vi "RT Communication Handler.vi"(8 "error in (no error)":errorcluster) -> (0 "error out":errorcluster)   [LabVIEW 2021]
uses:
  Controls/Communication Message Names.ctl
  Real-Time/Controls/Data FGV Action.ctl
  Controls/Scope & FGen Parameters.ctl
  Program Files (x86)/National Instruments/LabVIEW 2021/ProjectTemplates/Source/myRIO/Oscilloscope/myRIO v1.1/Real-Time/Controls/Wave Parameters.ctl
  Program Files (x86)/National Instruments/LabVIEW 2021/ProjectTemplates/Source/myRIO/Oscilloscope/myRIO v1.1/Real-Time/Controls/Waveform Enum.ctl
  Program Files (x86)/National Instruments/LabVIEW 2021/ProjectTemplates/Source/myRIO/Oscilloscope/myRIO v1.1/Real-Time/Controls/Channel Selector.ctl
  Controls/Time Selector.ctl
  Controls/Time Knob.ctl
  <vilib>/NI/STM/TCP/Write Meta Data (TCP Ref).vi
  <vilib>/NI/STM/TCP/Get Connection Reference (TCP).vi
  <vilib>/NI/STM/TCP/Write Meta Data (TCP Clst).vi
  <vilib>/NI/STM/TCP/Read Message (TCP).vi
  Real-Time/Controls/Global Stop.vi
  <vilib>/NI/STM/TCP/Write Message (TCP).vi
  <vilib>/NI/STM/NI STM.lvlib
panel:
  in  "Messages":T1=enum."New Settings"
  out "stop":bool
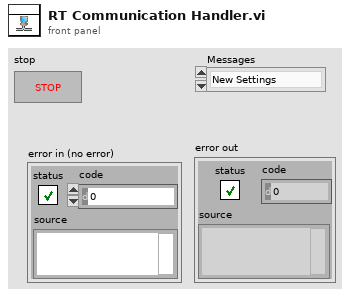
[diagram p1: front panel]
types:
  T1 = typedef "Communication Message Names.ctl" = enum16{"Status Check", "New Settings", "Measurements", "Acquire", "Params", "Initialize", "Stop"}
  T2 = typedef "Data FGV Action.ctl" = enum16{"Initialize", "Set Scope Data", "Read Scope Data", "Set FGen", "Read FGen", "Set Params"}
  T3 = typedef "Scope & FGen Parameters.ctl" = cluster{"Acquire?":bool, "Wave Parameters":T4, "Time":T7}
  T4 = typedef "Wave Parameters.ctl" = cluster{"Frequency (Hz)":dbl, "Phase offset (deg)":dbl, "Vpeak (V)":dbl, "Offset (V)":dbl, "Waveform":T5, "Channel":T6}
  T5 = typedef "Waveform Enum.ctl" = enum16{"Sine", "Square"}
  T6 = typedef "Channel Selector.ctl" = enum16{"CH0", "CH1"}
  T7 = typedef "Time Selector.ctl" = cluster{"Time/Div":T8}
  T8 = typedef "Time Knob.ctl" = dbl
  T9 = typedef "NI STM.lvlib/TCP Connection Info.ctl" = cluster{"connection ID":refnum<k5>, "meta data":T10[]}
  T10 = typedef "NI STM.lvlib/MetaDataElement.ctl" = string
  T11 = typedef "Scope Data.ctl" = cluster{"AI0":dbl[], "AI1":dbl[]}
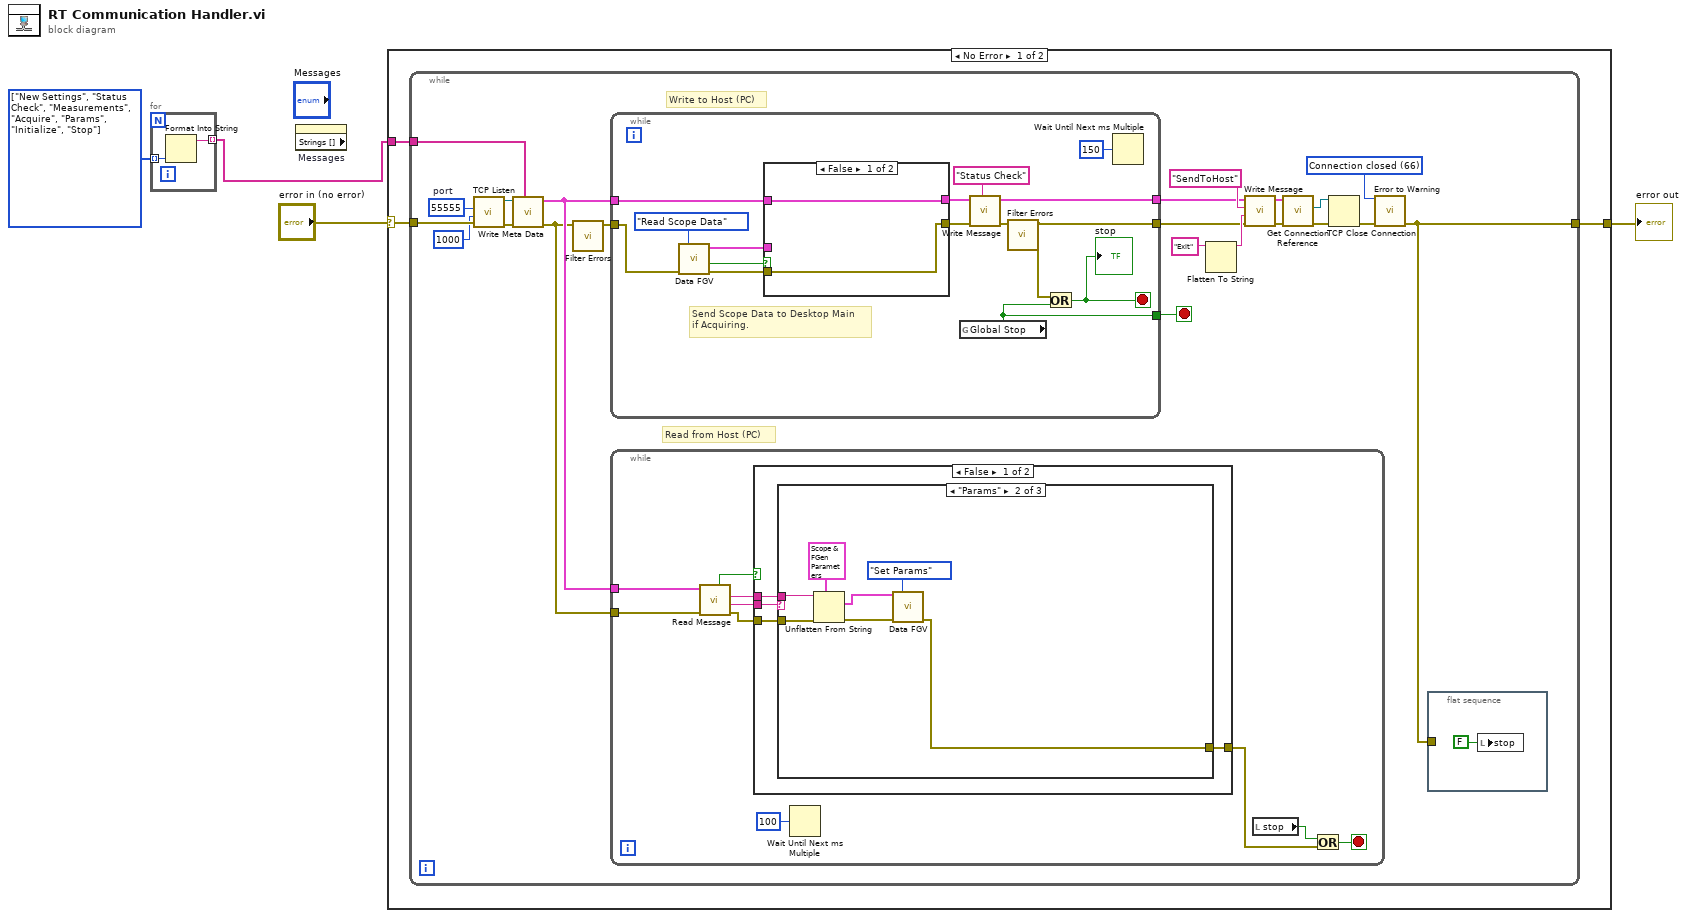
[diagram p0: block diagram]
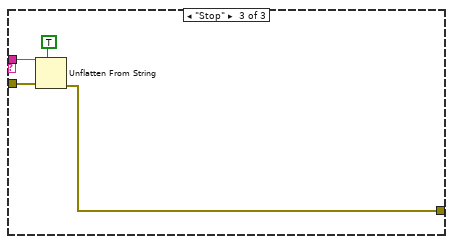
[diagram p3: hidden frame]
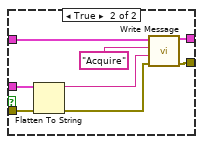
[diagram p5: hidden frame]
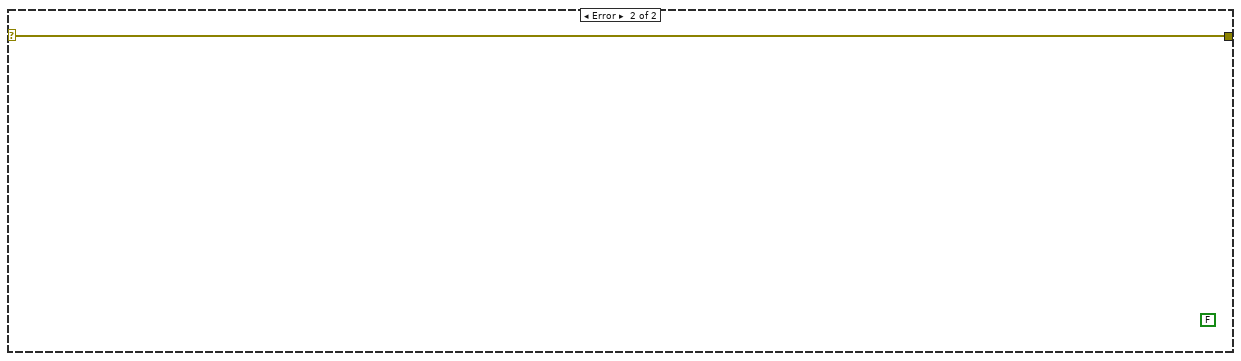
[diagram p6: hidden frame]
diagram:
  w2 = T1[] [enum."New Settings", enum."Status Check", enum."Measurements", enum."Acquire", enum."Params", enum."Initialize", enum."Stop"] items=["Status Check", "New Settings", "Measurements", "Acquire", "Params", "Initialize", "Stop"]
  n1 = for {
    tunnel: w2 -> [w6] mode=indexing
    tunnel: [w5] -> w1 mode=indexing
    n2 = Format Into String(w6) -> (resulting string=w5:string)  [unwired: 3 in, 1 out]
  }
  n3 = property on="Messages" class="Enum (strict)" props=["Strings []"]() -> ()  [unwired: 2 in, 3 out]
  n4 = case shown="No Error" "error in (no error)" {
    selector: "error in (no error)" -> [w8 w85]
    tunnel: [w9 w85] -> w4
    tunnel: w1 -> [w7 _]
    frame No Error {
      n5 = while {
        tunnel: [w23] -> w9
        tunnel: w8 -> [w22]
        tunnel: w7 -> [w14]
        stop <- w24 stop-if-true
        w26 = 66 items=["No Error", "Argument Error", "Memory Full", "Out of Zone", "End of File", "File Already Open", "Generic File IO Error", "File Not Found", "File Permission Error", "Disk Full", "Duplicate Path", "Too Many Files Open", "Not Enabled", "Resource File Not Found", "Cannot Add Resource", "Resource Not Found", "Image Not Found", "Image Memory Error", "Pen Does Not Exist", "Config Bad Type", "Config Token Not Found", "Config Parse Error", "Config Memory Error", "Bad External Code Format", "Bad External Code Offset", "External Code Not Present", "Null Window", "Destroy Window Mixup", "Null Menu", "Print Aborted", "Bad Print Record", "Print Driver Error", "Windows Error During Print", "Memory Error During Print", "Print Dialog Error", "Generic Print Error", "Invalid Device Refnum", "Device Not Found", "Device Parameter Error", "Device Unit Error", "Can't Open Device", "Device Call Aborted", "Generic Error", "Cancelled By User", "Object ID Too Low", "Object ID Too High", "Object Not In Heap", "Unknown Heap", "Bad DefProc ID", "DefProc Not In Table", "Message Out Of Range", "Null Method", "Unknown Message", "Manager Call Not Supported", "Bad address", "Connection In progress", "Connection timed out", "Connection is already in progress", "Network attribute not supported", "Network error", "Address in use", "System out of memory", "Connection aborted", "Connection refused", "Connection is not connected", "Connection is already connected", "Connection closed", "Initialize error (interapplication manager)", "Bad occurrence", "Wait on unbound occurrence handler", "Occurrence queue overflow", "Bad path", "Semaphore not signaled", "Unrecognized type (interapplication manager)"] ("1st Error to Convert")
        w31 = u16 55555  # port
        # "Read from Host (PC)"
        # "Write to Host (PC)"
        n6 = call <vilib>:"TCP Listen.vi"("error in (no error)"=w22, "timeout ms (wait forever: -1)"=1000, "port"=w31) -> ("error out"=w29:errorcluster, "connection ID"=w30:refnum<k5>)  [unwired: 1 in, 6 out]
        n7 = call-poly <vilib>:"Write Meta Data.vi"("meta data"=w14, "error in"=w29, "connection ID"=w30) -> ("error out"=w10:errorcluster, "connection info out"=w15:T9)  [unwired: 2 in, 5 out]
        n8 = call "Filter Errors.vi"("error in (no error)"=w10) -> ("error out"=w11:errorcluster)  [unwired: 10 in]
        n9 = while {
          tunnel: w11 -> [w72]
          tunnel: w15 -> [w74]
          tunnel: [w61] -> w17
          tunnel: [w64] -> w16
          tunnel: [w62] -> w24
          stop <- w67 stop-if-true
          # "Send Scope Data to Desktop Main\nif Acquiring."
          n10 = call "Data FGV.vi"("Action"=Data_FGV_Action."Read Scope Data", "error in (no error)"=w72) -> ("Scope Data"=w69:T11, "Acquire?"=w68:bool, "error out"=w70:errorcluster)  [unwired: 9 in, 2 out]
          n11 = case shown="False" w68 {
            tunnel: w74 -> [w76 w84]
            tunnel: [w76 w83] -> w65
            tunnel: [w75 w82] -> w66
            tunnel: w70 -> [w75 w81]
            tunnel: w69 -> [_ w78]
            frame False {
            }
            frame True {
              n12 = Flatten To String(anything=w78, error in (no error)=w81) -> (data string=w79:string, error out=w80:errorcluster)  [unwired: 2 in, 1 out]
              n13 = call-poly <vilib>:"Write Message.vi"("error in"=w80, "data"=w79, "name"="Acquire", "connection info in"=w84) -> ("error out"=w82:errorcluster, "connection info out"=w83:T9)  [unwired: 1 in, 5 out]
            }
          }
          n14 = global read "Global Stop.vi" "Global Stop"() -> (w62:bool)
          n15 = call-poly <vilib>:"Write Message.vi"("error in"=w66, "name"="Status Check", "connection info in"=w65) -> ("error out"=w60:errorcluster, "connection info out"=w64:T9)  [unwired: 2 in, 5 out]
          n16 = call "Filter Errors.vi"("error in (no error)"=w60) -> ("error out"=w61:errorcluster)  [unwired: 10 in]
          n17 = Or(x=w61, y=w62) -> (x .or. y?=w67:bool)
          "stop" <- w67
          n18 = Wait Until Next ms Multiple(millisecond multiple=u32 150) -> ()  [unwired: 1 out]
        }
        n19 = while {
          tunnel: w15 -> [w42]
          tunnel: w10 -> [w33]
          stop <- w38 stop-if-true
          n20 = call-poly <vilib>:"Read Message.vi"("error in"=w33, "connection info in"=w42) -> ("error out"=w36:errorcluster, "name"=w40:T10, "data string"=w39:string, "timed out?"=w41:bool)  [unwired: 4 in, 2 out]
          n21 = case shown="False" w41 {
            tunnel: w40 -> [w46 _]
            tunnel: w39 -> [w45 _]
            tunnel: w36 -> [w44 w59]
            tunnel: [w43 w59] -> w35
            frame False {
              n22 = case shown="\"Params\"" w46 {
                tunnel: w45 -> [_ w53 w57]
                tunnel: w44 -> [w47 w54 w58]
                tunnel: [w47 w48 w55] -> w43
                frame "False", Default {
                }
                frame "Params" {
                  n23 = Unflatten From String(type=T3 {"Acquire?"=FALSE, "Wave Parameters"={"Frequency (Hz)"=5.0, "Phase offset (deg)"=0.0, "Vpeak (V)"=5.0, "Offset (V)"=0.0, "Waveform"=enum."Sine", "Channel"=enum."CH0"}, "Time"={"Time/Div"=0.0}} ("Params"), binary string=w53, error in (no error)=w54) -> (value=w51:T3, error out=w49:errorcluster)  [unwired: 2 in, 1 out]
                  n24 = call "Data FGV.vi"("Params"=w51, "Action"=Data_FGV_Action."Set Params", "error in (no error)"=w49) -> ("error out"=w48:errorcluster)  [unwired: 8 in, 4 out]
                }
                frame "Stop" {
                  n25 = Unflatten From String(type=TRUE, binary string=w57, error in (no error)=w58) -> (error out=w55:errorcluster)  [unwired: 2 in, 2 out]
                }
              }
            }
            frame True {
            }
          }
          n26 = Wait Until Next ms Multiple(millisecond multiple=u32 100) -> ()  [unwired: 1 out]
          n27 = local read "stop"() -> (w34:bool)
          n28 = Or(x=w34, y=w35) -> (x .or. y?=w38:bool)
        }
        n29 = Flatten To String(anything="Exit") -> (data string=w20:string)  [unwired: 1 in, 4 out]
        n30 = call-poly <vilib>:"Write Message.vi"("error in"=w17, "data"=w20, "name"="SendToHost" ("Name"), "connection info in"=w16) -> ("error out"=w18:errorcluster, "connection info out"=w19:T9)  [unwired: 2 in, 4 out]
        n31 = call-poly <vilib>:"Get Connection Reference.vi"("error in"=w18, "connection info in"=w19) -> ("error out"=w27:errorcluster, "connection ID out"=w28:refnum<k5>)  [unwired: 8 out]
        n32 = TCP Close Connection(connection ID=w28, error in (no error)=w27) -> (error out=w25:errorcluster)  [unwired: 2 out]
        n33 = call <vilib>:"Error to Warning.vi"("1st Error to Convert"=w26, "error in"=w25) -> ("warning out"=w23:errorcluster)  [unwired: 3 in, 10 out]
        n34 = flat-sequence {
          tunnel: w23 -> [_]
          frame #0 {
            n35 = local write "stop"(FALSE ("stop")) -> ()
          }
        }
      }
    }
    frame Error {
      (unwired) FALSE ("Restart")
    }
  }
  "error out" <- w4
